vi "programacion 11 parcial 2.vi"() -> ()   [LabVIEW 2011]
uses:
  control de programacion 11 parcial 2.ctl
panel:
  out "Array":dbl[][](array[numeric])
  # "Ingresar numeros enteros entre 1-200, luego en la ultima del arreglo \nreservarla para obtener el numero mayor de cada una de las columnas."
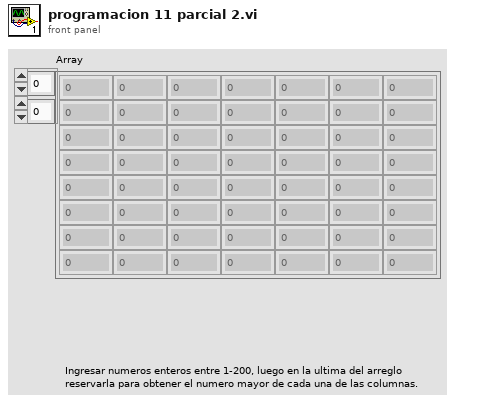
[diagram p1: front panel]
types:
  T1 = typedef "control de programacion 11 parcial 2.ctl" = enum16{"inicializar", "rellenar", "mayor numero", "finalizar"}
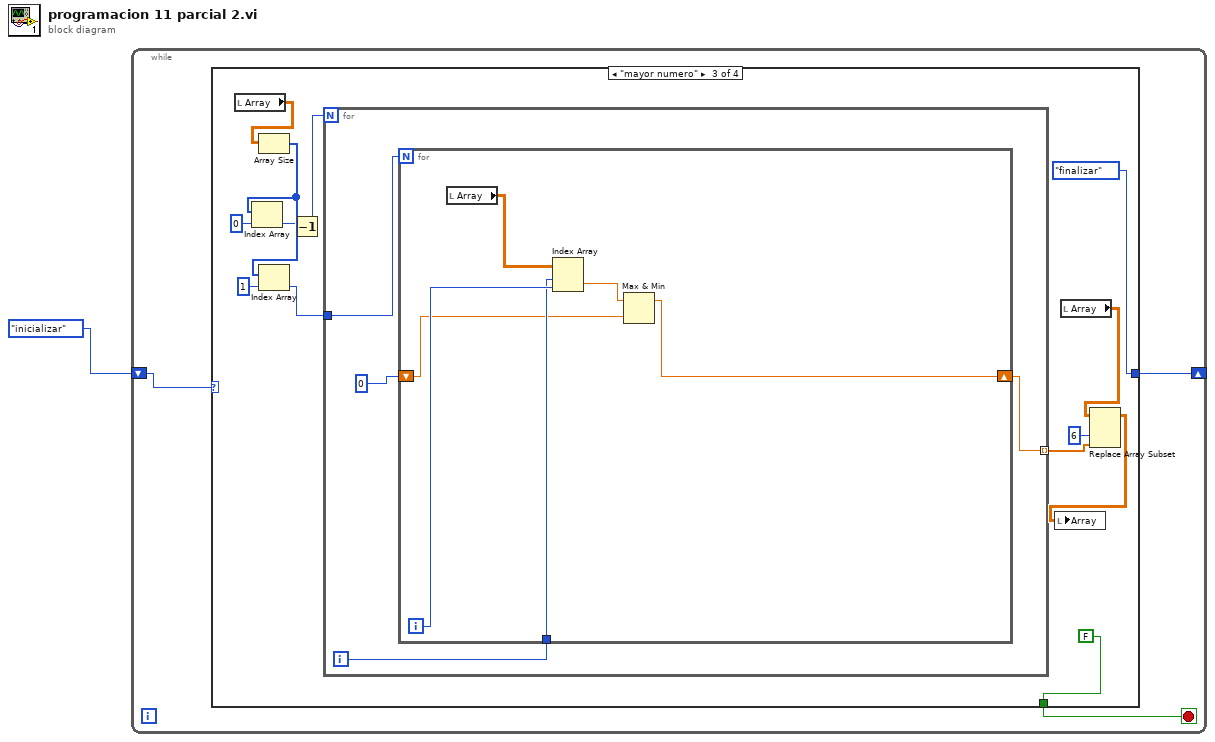
[diagram p0: block diagram]
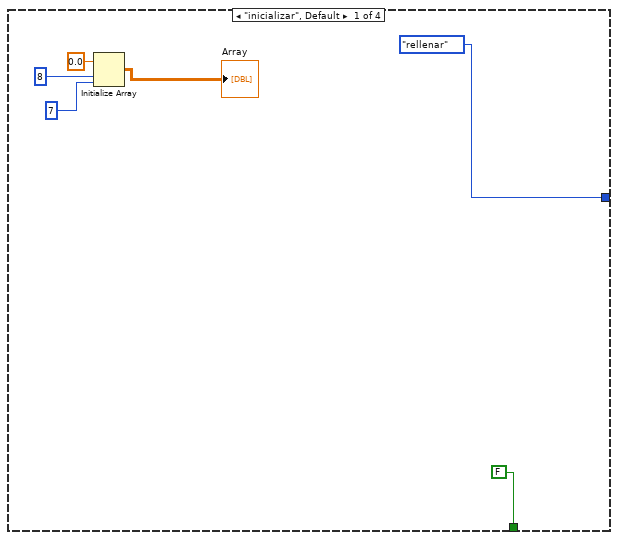
[diagram p2: hidden frame]
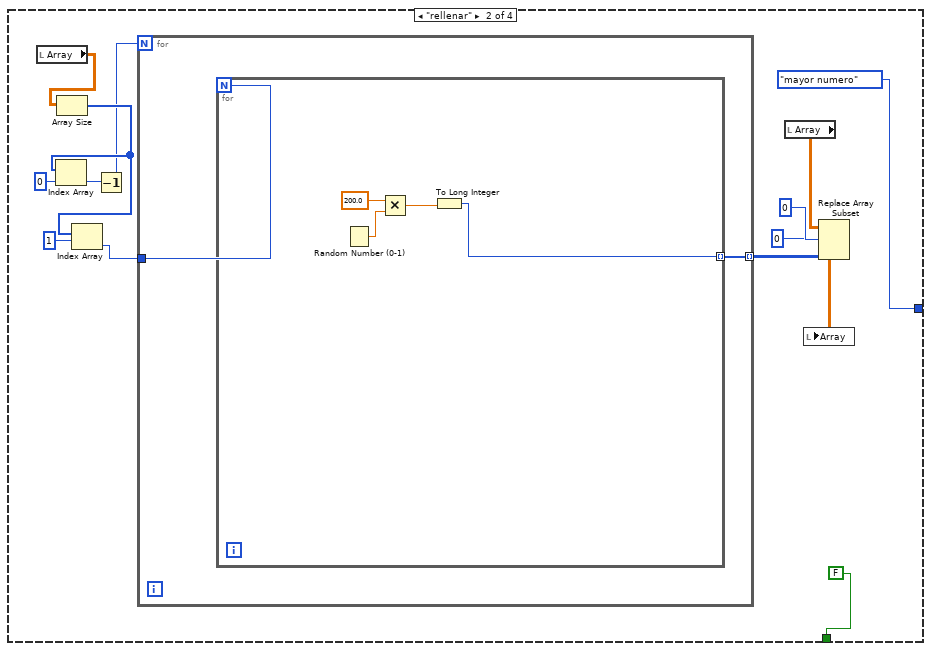
[diagram p3: hidden frame]
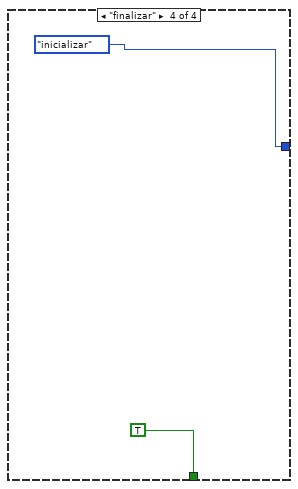
[diagram p4: hidden frame]
diagram:
  n1 = while {
    shift-right: [w3] -> _
    shift-left: control_de_programacion_11_parcial_2."inicializar" -> [w4]
    stop <- w2 stop-if-true
    n2 = case shown="\"mayor numero\"" w4 {
      tunnel: [control_de_programacion_11_parcial_2."rellenar" control_de_programacion_11_parcial_2."mayor numero" control_de_programacion_11_parcial_2."finalizar" control_de_programacion_11_parcial_2."inicializar"] -> w3
      tunnel: [FALSE FALSE FALSE TRUE] -> w2
      frame "inicializar", Default {
        n3 = Initialize Array(0.0 ("element"), 8 ("dimension size"), 7 ("dimension size")) -> (→"Array":dbl[][])
      }
      frame "rellenar" {
        n4 = local read "Array"() -> (w21:dbl[][])
        n5 = Array Size(array=w21) -> (size(s)=w23:i32[])
        n6 = Index Array(array=w23, index=0) -> (element=w13:i32)
        n7 = Index Array(array=w23, index=1) -> (element=w11:i32)
        n8 = Decrement(x=w13) -> (x-1=w12:i32)
        n9 = for {
          N: w12 -> [_]
          tunnel: w11 -> [w26]
          tunnel: [w25] -> w17 mode=indexing
          n10 = for {
            N: w26 -> [_]
            tunnel: [w27] -> w25 mode=indexing
            n11 = Random Number (0-1)() -> (number: 0 to 1=w29:dbl)
            n12 = Multiply(x=200.0, y=w29) -> (x*y=w28:dbl)
            n13 = To Long Integer(number=w28) -> (32bit integer=w27:i32)
          }
        }
        n14 = local read "Array"() -> (w20:dbl[][])
        n15 = Replace Array Subset(array=w20, new element=w17, index (row)=0, index (col)=0 ("disabled index (col)")) -> (w16:dbl[][])
        n16 = local write "Array"(w16) -> ()
      }
      frame "mayor numero" {
        n17 = local read "Array"() -> (w43:dbl[][])
        n18 = Array Size(array=w43) -> (size(s)=w41:i32[])
        n19 = Index Array(array=w41, index=0) -> (element=w33:i32)
        n20 = Index Array(array=w41, index=1) -> (element=w31:i32)
        n21 = Decrement(x=w33) -> (x-1=w32:i32)
        n22 = for {
          N: w32 -> [_]
          tunnel: w31 -> [w47]
          tunnel: [w44] -> w37 mode=indexing
          i -> [w46]
          n23 = for {
            N: w47 -> [_]
            tunnel: w46 -> [w51]
            shift-right: [w48] -> w44
            shift-left: 0 -> [w49]
            i -> [w52]
            n24 = local read "Array"() -> (w53:dbl[][])
            n25 = Index Array(array=w53, index (row)=w51, index (col)=w52) -> (element=w50:dbl)
            n26 = Max & Min(x=w50, y=w49) -> (max(x,y)=w48:dbl)  [unwired: 1 out]
          }
        }
        n27 = local read "Array"() -> (w39:dbl[][])
        n28 = Replace Array Subset(array=w39, new element=w37, index (col)=6 ("disabled index (col)")) -> (w36:dbl[][])  [unwired: 1 in]
        n29 = local write "Array"(w36) -> ()
      }
      frame "finalizar" {
      }
    }
  }
